vi "ConstrainedState_SetVelocity.vi"(10 "maxVelocity":dbl, 11 "inCONSTRAINED_STATE":T1={"POSEwCURVATURE"={"CURVATURE"=0.0, "POSE"={"TRANSLATION"={"X"=0.0, "Y"=0.0}, "ROTATION"={"VALUE"=0.0, "COS"=1.0, "SIN"=0.0}}}, "Distance"=0.0, "minAccel"=0.0, "maxAccel"=0.0, "maxVelocity"=0.0} {"POSEwCURVATURE"."POSE"."ROTATION"."SIN" format="%13.4f"; "POSEwCURVATURE"."POSE"."ROTATION"."COS" format="%13.4f"; "POSEwCURVATURE"."POSE"."ROTATION"."VALUE" format="%13.4f"; "POSEwCURVATURE"."POSE"."TRANSLATION"."Y" format="%14.3f"; "POSEwCURVATURE"."POSE"."TRANSLATION"."X" format="%14.3f"}) -> (3 "outCONSTRAINED_STATE":T1={"POSEwCURVATURE"={"CURVATURE"=0.0, "POSE"={"TRANSLATION"={"X"=0.0, "Y"=0.0}, "ROTATION"={"VALUE"=0.0, "COS"=1.0, "SIN"=0.0}}}, "Distance"=0.0, "minAccel"=0.0, "maxAccel"=0.0, "maxVelocity"=0.0} {"POSEwCURVATURE"."POSE"."ROTATION"."SIN" format="%13.4f"; "POSEwCURVATURE"."POSE"."ROTATION"."COS" format="%13.4f"; "POSEwCURVATURE"."POSE"."ROTATION"."VALUE" format="%13.4f"; "POSEwCURVATURE"."POSE"."TRANSLATION"."Y" format="%14.3f"; "POSEwCURVATURE"."POSE"."TRANSLATION"."X" format="%14.3f"})   [LabVIEW 2019, in "Trajectory_Library.lvlib"]
doc: "Internal routine used only by TrajectoryParam_timeParam."
uses:
  Trajectory_Library.lvlib
  TypeDef/TRANSLATION2D.ctl
  TypeDef/ROTATION2D.ctl
  TypeDef/POSEwCURVATURE.ctl
  TypeDef/POSE2D.ctl
  TypeDef/CONSTRAINED_STATE.ctl
panel:
  # "All units\nare SI"
  # "All units\nare SI"
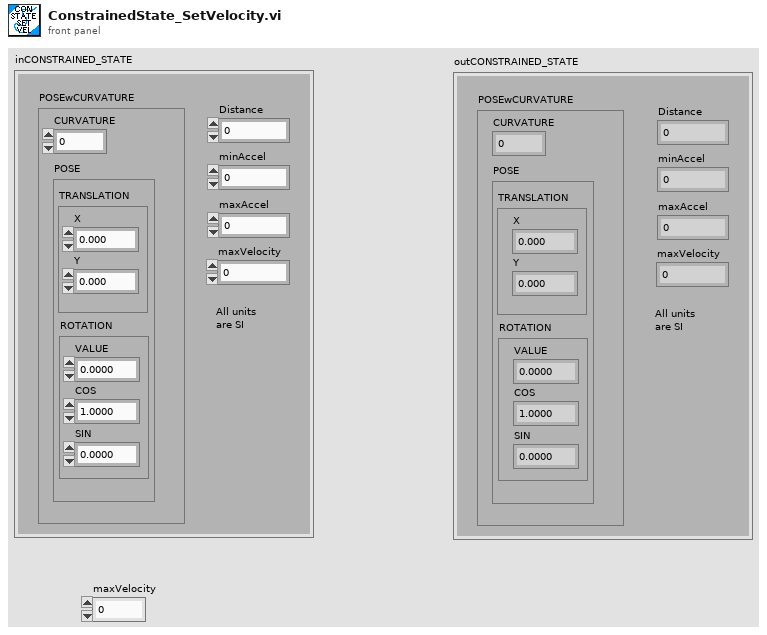
[diagram p1: front panel]
types:
  T1 = typedef "Trajectory_Library.lvlib/CONSTRAINED_STATE.ctl" = cluster{"POSEwCURVATURE":T2, "Distance":dbl, "minAccel":dbl, "maxAccel":dbl, "maxVelocity":dbl}
  T2 = typedef "Trajectory_Library.lvlib/POSEwCURVATURE.ctl" = cluster{"CURVATURE":dbl, "POSE":T3}
  T3 = typedef "Trajectory_Library.lvlib/POSE2D.ctl" = cluster{"TRANSLATION":T4, "ROTATION":T5}
  T4 = typedef "Trajectory_Library.lvlib/TRANSLATION2D.ctl" = cluster{"X":dbl, "Y":dbl}
  T5 = typedef "Trajectory_Library.lvlib/ROTATION2D.ctl" = cluster{"VALUE":dbl, "COS":dbl, "SIN":dbl}
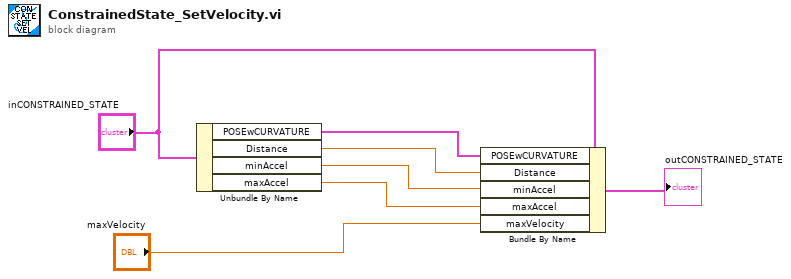
[diagram p0: block diagram]
diagram:
  n1 = Unbundle By Name("inCONSTRAINED_STATE") -> ("POSEwCURVATURE"=w4:T2, "Distance"=w3:dbl, "minAccel"=w2:dbl, "maxAccel"=w1:dbl)
  n2 = Bundle By Name(cluster="inCONSTRAINED_STATE", "POSEwCURVATURE"=w4, "Distance"=w3, "minAccel"=w2, "maxAccel"=w1, "maxVelocity"="maxVelocity") -> (→"outCONSTRAINED_STATE":T1)
